vi "Reduced Density Matrix.vi"(7 "QuWires Array":refnum<class "QuWire.lvclass">[](array[class])) -> (8 "Density Matrix (Reduced)":cdb[][](array[numeric]))   [LabVIEW 2020]
uses:
  QuSim/QuWire/QuWire.lvclass
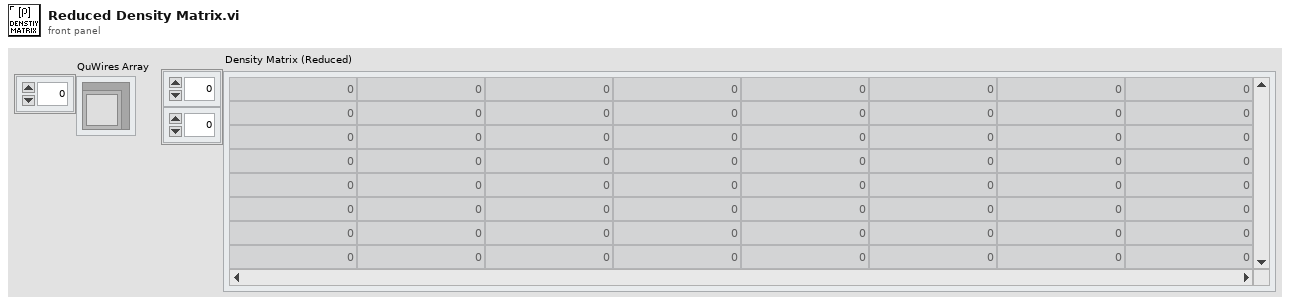
[diagram p1: front panel]
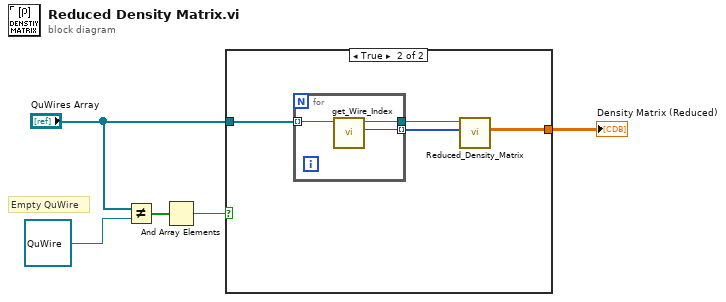
[diagram p0: block diagram]
diagram:
  # "Empty QuWire"
  n1 = Not Equal?(x="QuWires Array", y=refnum<class "QuWire.lvclass"> refnum ("QuWire in")) -> (x != y?=w4:bool[])
  n2 = And Array Elements(Boolean array=w4) -> (logical AND=w5:bool)
  n3 = case shown="True" w5 {
    tunnel: "QuWires Array" -> [_ w8]
    tunnel: [_ w9] -> w1
    frame False {
    }
    frame True {
      n4 = for {
        tunnel: w8 -> [w12] mode=indexing
        tunnel: [w11] -> w7
        tunnel: [w10] -> w6 mode=indexing
        n5 = call "get_Wire_Index.vi"("QuWire in"=w12) -> ("Wire Index"=w10:i32, "QuWire out"=w11:refnum<class "QuWire.lvclass">)  [unwired: 8 in, 1 out]
      }
      n6 = call "Reduced_Density_Matrix.vi"("Qubits to Keep"=w6, "QuWire in"=w7) -> ("Reduced Density Matrix"=w9:cdb[][])  [unwired: 7 in, 2 out]
    }
  }
  "Density Matrix (Reduced)" <- w1
